vi "Init.vi"(8 "error in (no error)":errorcluster, 11 "Data":variant) -> (0 "error out":errorcluster)   [LabVIEW 2018, in "Error Handler.lvlib"]
doc: "This subVI enqueues the named action in to the communications queue along with the input data."
uses:
  Error Handler.lvlib
  Private Controls/Module Data.ctl
  Private Controls/Module Action.ctl
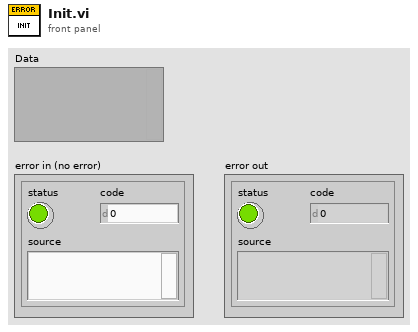
[diagram p1: front panel]
types:
  T1 = typedef "Error Handler.lvlib/Module Data.ctl" = cluster{"Data":variant, "Action":T2}
  T2 = typedef "Error Handler.lvlib/Module Action.ctl" = enum8{"Init", "Exit", "Controller Error", "UI1 Error", "UI2 Error", "UI3 Error", "File IO Error", "cRIO Error", "Calibration Error"}
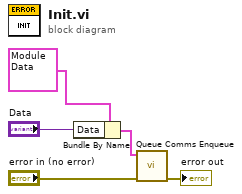
[diagram p0: block diagram]
diagram:
  n1 = Bundle By Name(cluster=T1 {"Data"=variant, "Action"=enum."Init"} ("element"), "Data"="Data") -> (w4:T1)
  n2 = call "Queue Comms Enqueue.vi"("error in (no error)"="error in (no error)", "element"=w4) -> ("error out"=→"error out":errorcluster)  [unwired: 9 in]
